vi "kpro 2016.vi"(0 "Output KPRO":path=path "c:/junk.dat", 1 "Initialize":bool, 2 "Finished In":bool, 3 "Cluster":T2, 5 "Absolute Depth In":sgl format="%.2f", 7 "Sensor Cluster In":T1, 11 "Flow":dbl format="%.2f", 12 "Read String Pot":bool, 13 "Increment":bool, 14 "SS In":i32) -> (4 "Finished Out":bool, 6 "SS Out":i32, 8 "Current Depth Out":sgl format="%.2f", 15 "Output Array":dbl[][](array[numeric])=[[17182499.0, -1.0, -1.0, 0.07295542423579193, 10.0, 30.0, 1.0, 0.2942041776993234, 33.989999999999995], [17194122.0, -2.0, -2.0, 0.08603630732168976, 10.0, 30.0, 1.0, 0.28579594169762795, 34.989999999999995], [17196835.0, -3.0, -3.0, 0.36859565057132326, 10.0, 30.0, 1.0, 0.27785495971103086, 35.989999999999995], [17198861.0, -4.0, -4.0, 0.493583415597236, 10.0, 30.0, 1.0, 0.27034333603676675, 36.989999999999995], [17203069.0, -5.0, -5.0, 0.23764258555133078, 10.0, 30.0, 1.0, 0.2632271650434325, 37.989999999999995], [17204351.0, -6.0, -6.0, 0.7800312012480499, 10.0, 30.0, 1.0, 0.2564760194921775, 38.989999999999995], [17205734.0, -7.0, -7.0, 0.7230657989877078, 10.0, 30.0, 1.0, 0.25006251562890724, 39.989999999999995], [17206879.0, -8.0, -8.0, 0.8733624454148472, 10.0, 30.0, 1.0, 0.24396194193705784, 40.989999999999995], [17208211.0, -9.0, -9.0, 0.7507507507507507, 10.0, 30.0, 1.0, 0.23815194093831868, 41.989999999999995], [17211804.0, -10.0, -10.0, 0.27831895352073477, 10.0, 30.0, 1.0, 0.23261223540358225, 42.989999999999995], [17214313.0, -11.0, -11.0, 0.3985651654045437, 10.0, 30.0, 1.0, 0.22732439190725168, 43.989999999999995], [17215593.0, -12.0, -12.0, 0.78125, 10.0, 30.0, 1.0, 0.22227161591464772, 44.989999999999995], [17216822.0, -13.0, -13.0, 0.8136696501220504, 10.0, 30.0, 1.0, 0.21743857360295718, 45.989999999999995], [17218103.0, -14.0, -14.0, 0.7806401249024201, 10.0, 30.0, 1.0, 0.2128112364332837, 46.989999999999995], [17219267.0, -15.0, -15.0, 0.859106529209622, 10.0, 30.0, 1.0, 0.20837674515524068, 47.989999999999995], [17220448.0, -16.0, -16.0, 0.8467400508044031, 10.0, 30.0, 1.0, 0.20412329046744235, 48.989999999999995], [17221627.0, -17.0, -17.0, 0.8481764206955046, 10.0, 30.0, 1.0, 0.20004000800160035, 49.989999999999995], [17222775.0, -18.0, -18.0, 0.8710801393728224, 10.0, 30.0, 1.0, 0.19611688566385568, 50.989999999999995], [17223888.0, -19.0, -19.0, 0.8984725965858041, 10.0, 30.0, 1.0, 0.19234468166955185, 51.989999999999995], [17225019.0, -20.0, -20.0, 0.8841732979664014, 10.0, 30.0, 1.0, 0.18871485185884132, 52.989999999999995], [17226151.0, -21.0, -21.0, 0.88339222614841, 10.0, 30.0, 1.0, 0.18521948508983146, 53.989999999999995], [17227282.0, -22.0, -22.0, 0.8841732979664014, 10.0, 30.0, 1.0, 0.18185124568103292, 54.989999999999995]] format="%.5f")   [LabVIEW 2016]
uses:
  controls/Kpro hydraulic measurement cluster.ctl
  controls/MCC DAQ Readings.ctl
  C:/Cascade-lv16-64/builds/Waterloo Main Program/cascade/data/ULx_LV.dll
  builds/Waterloo Main Program/cascade/data/ULx_LV.dll
panel:
  out "Sensor Cluster 2":T1
  in  "Sensor Cluster In 2":T1
  out "Array out":refnum<k24>[](array[refnum])
  in  "Array in":refnum<k24>[](array[refnum])
  in  "String Pot \nSlope 2":dbl=1.7339999675750732 format="%.2f"
  in  "error in (no error)":errorcluster
  in  "Descriptions":string[](array[string])
  in  "Output KPRO 2":path=path "c:/junk.dat"
  in  "Zeroed Pressure 2":dbl format="%.2f"
  out "Cluster Out":T2
  in  "String Pot \nSlope":dbl=1.7339999675750732 format="%.2f"
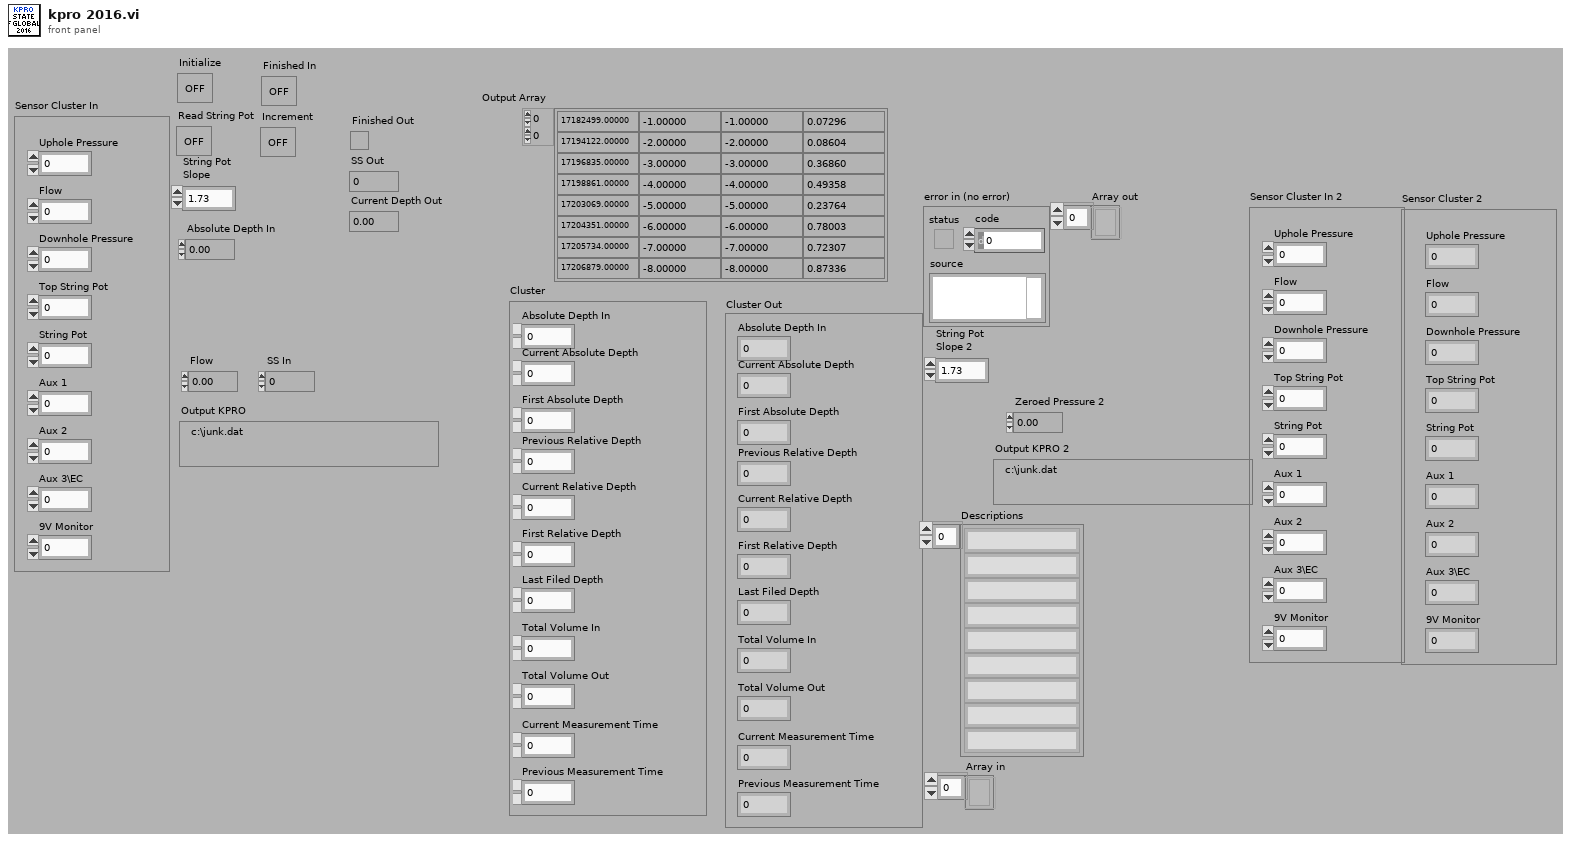
[diagram p1: front panel]
types:
  T1 = typedef "MCC DAQ Readings.ctl" = cluster{"Uphole Pressure":dbl, "Flow":dbl, "Downhole Pressure":dbl, "Top String Pot":dbl, "String Pot":dbl, "Aux 1":dbl, "Aux 2":dbl, "Aux 3\\EC":dbl, "9V Monitor":dbl}
  T2 = typedef "Kpro hydraulic measurement cluster.ctl" = cluster{"Absolute Depth In":dbl, "Current Absolute Depth":dbl, "First Absolute Depth":dbl, "Previous Relative Depth":dbl, "Current Relative Depth":dbl, "First Relative Depth":dbl, "Last Filed Depth":dbl, "Total Volume In":dbl, "Total Volume Out":dbl, "Current Measurement Time":dbl, "Previous Measurement Time":dbl}
  T3 = enum16{"Initialize", "Read", "Calc IK and generate Array", "Write Data & finish"}
  T4 = enum16{"Initialize", "Read", "read2", "Write Data & finish"}
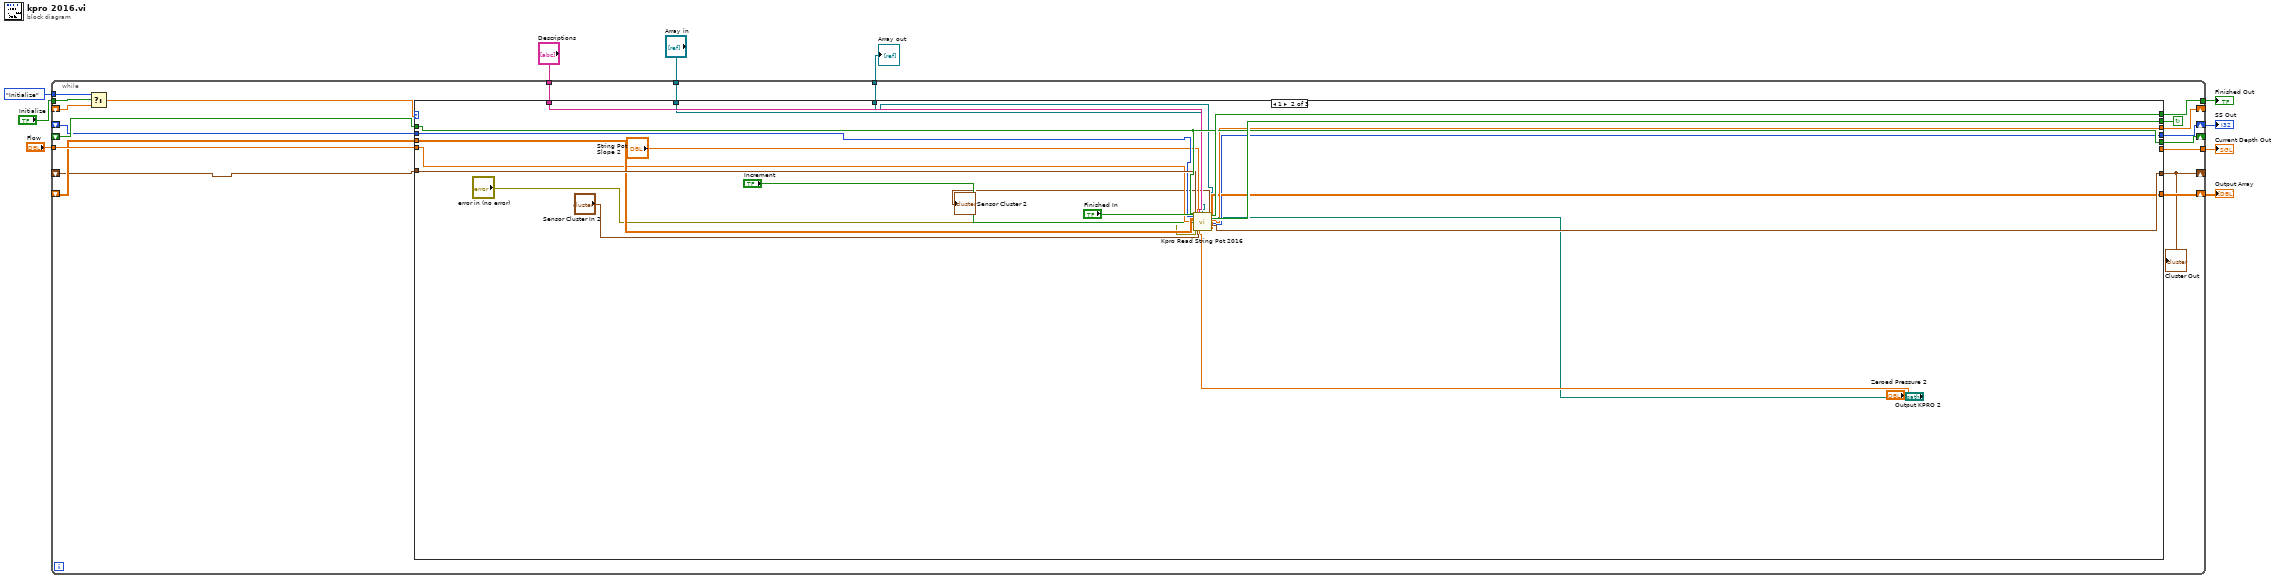
[diagram p0: block diagram]
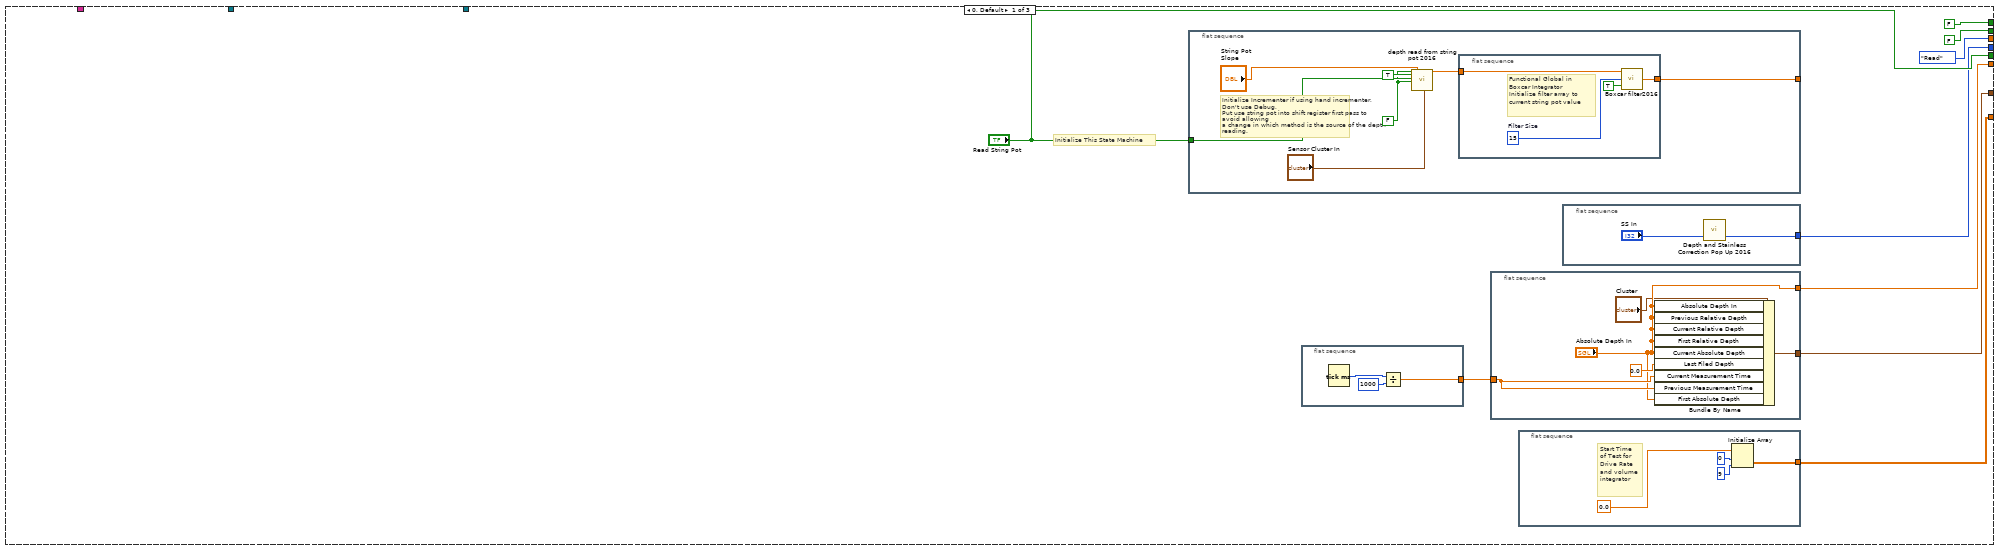
[diagram p2: hidden frame]
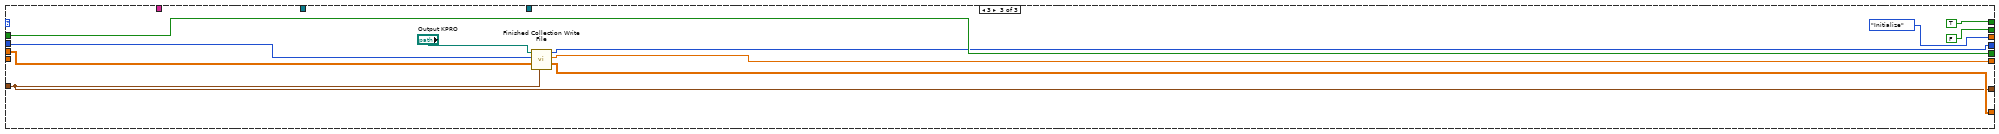
[diagram p3: hidden frame]
diagram:
  n1 = while {
    shift-left: _ -> [w22]
    shift-right: [w21] -> w5
    tunnel: [w23] -> w6
    tunnel: [w24] -> w7
    shift-left: _ -> [w25]
    shift-right: [w26] -> w4
    tunnel: "Flow" -> [w27]
    shift-left: _ -> [w28]
    shift-right: [w29] -> _
    tunnel: "Initialize" -> [w30]
    tunnel: T3."Initialize" -> [w19]
    shift-left: _ -> [w17]
    shift-right: [w16] -> _
    shift-right: [w15] -> _
    shift-left: _ -> [w14]
    tunnel: "Descriptions" -> [w13]
    tunnel: [w12] -> w2
    tunnel: "Array in" -> [w11]
    stop <- w20 continue-if-true
    n2 = Select(t=w19, s=w30, f=w17) -> (s? t:f=w18:dbl)
    n3 = case shown="1" w18 {
      tunnel: [T4."Read" w80 T3."Initialize"] -> w16
      tunnel: ["Read String Pot" w83 w96] -> w29
      tunnel: w28 -> [_ w83 w96]
      tunnel: w27 -> [_ w76 _]
      tunnel: [w38 w78 w93] -> w26
      tunnel: w25 -> [_ w79 w95]
      tunnel: [w31 _ w94] -> w24
      tunnel: [FALSE w86 FALSE] -> w20
      tunnel: [FALSE w84 TRUE] -> w23
      tunnel: w22 -> [_ w77 w91]
      tunnel: [w35 w75 w90] -> w21
      tunnel: [w33 w81 w88] -> w15
      tunnel: w14 -> [_ w82 w88]
      tunnel: w13 -> [_ w74 _]
      tunnel: [_ w73 _] -> w12
      tunnel: w11 -> [_ w72 _]
      frame 0, Default {
        # "Initialize This State Machine"
        n4 = flat-sequence {
          tunnel: "Read String Pot" -> [w54]
          tunnel: [w52] -> _
          frame #0 {
            w53 = FALSE
            # "Initialize Incrementer if using hand incrementer,\nDon't use Debug,\nPut use string pot into shift register first pass to avoid allowing\na change in which method is the source of the depth reading."
            n5 = call "depth read from string pot 2016.vi"(0:w53, 1:TRUE, 2:w54, 3:w53, "String Pot \nSlope"="String Pot \nSlope", "Sensor Cluster In"="Sensor Cluster In") -> ("Depth"=w56:dbl)  [unwired: 10 in, 3 out]
            n6 = flat-sequence {
              tunnel: w56 -> [w58]
              tunnel: [w57] -> w52
              frame #0 {
                w59 = 15  # Filter Size
                # "Functional Global in \nBoxcar Integrator\nInitialize filter array to \ncurrent string pot value"
                n7 = call "Boxcar filter2016.vi"("Initialize"=TRUE, "Filter Size"=w59, "Filter Input"=w58) -> ("Filter Output"=w57:dbl)
              }
            }
          }
        }
        n8 = flat-sequence {
          tunnel: [w47] -> w32
          frame #0 {
            n9 = Tick Count (ms)() -> (millisecond timer value=w49:u32)
            n10 = Divide(x=w49, y=u32 1000) -> (x/y=w47:dbl)
          }
        }
        n11 = flat-sequence {
          tunnel: [w46] -> w33
          tunnel: w32 -> [w44]
          tunnel: ["Absolute Depth In"] -> w31
          frame #0 {
            n12 = Bundle By Name(cluster="Cluster", "Absolute Depth In"="Absolute Depth In", "Previous Relative Depth"="Absolute Depth In", "Current Relative Depth"="Absolute Depth In", "First Relative Depth"="Absolute Depth In", "Current Absolute Depth"="Absolute Depth In", "Last Filed Depth"=0.0, "Current Measurement Time"=w44, "Previous Measurement Time"=w44, "First Absolute Depth"="Absolute Depth In") -> (w46:T2)
          }
        }
        n13 = flat-sequence {
          tunnel: [w64] -> w38
          frame #0 {
            # "Start Time\nof Test for\nDrive Rate\nand volume\nintegrator"
            n14 = Initialize Array(0.0, 0, 9) -> (w64:dbl[][])
          }
        }
        n15 = flat-sequence {
          tunnel: [w40] -> w35
          frame #0 {
            n16 = call "Depth and Stainless Correction Pop Up 2016.vi"("New Number\n of Stainless\n(Count)"="SS In") -> ("Feet of\nStainless to be\nUsed (Count)"=w40:i32)  [unwired: 1 in, 1 out]
          }
        }
      }
      frame 1 {
        n17 = call "Kpro Read String Pot 2016.vi"("Read String Pot"=w83, "Feet of\nStainless to be\nUsed (Count) in"=w77, "Session Array in"=w79, "Flow"=w76, "Manual Depth In"="Increment", "Finished In"="Finished In", "Depth Cluster in"=w82, "error in (no error)"="error in (no error)", "String Pot \nSlope in"="String Pot \nSlope 2", "Sensor Cluster In in"="Sensor Cluster In 2", "Descriptions"=w74, "Pressure in"="Zeroed Pressure 2", "Array in"=w72, "Initial Measurement Input"="Output KPRO 2") -> ("Sensor Cluster 2"=→"Sensor Cluster 2":T1, "Array out"=w73:refnum<k24>[], "Generate Array Calc IK"=w84:bool, "Finish Take Data"=w86:bool, "Depth Rate"=w80:dbl, "Feet of\nStainless to be\nUsed (Count) out"=w75:i32, "Depth Cluster out"=w81:T2, "Single String Pot Session Array out"=w78:dbl[][])  [unwired: 3 in, 3 out]
      }
      frame 3 {
        n18 = call "Finished Collection Write File.vi"("Cluster in"=w88, "Corrected Array in"=w95, "Feet of\nStainless to be\nUsed (Count) in"=w91, "Output KPRO"="Output KPRO") -> ("Corrected Array out"=w93:dbl[][], "Depth to \nbe Used \n(Feet)"=w94:sgl, "Feet of\nStainless to be\nUsed (Count) out"=w90:i32)  [unwired: 5 in]
      }
    }
    "Cluster Out" <- w15
  }
  "Current Depth Out" <- w7
  "Finished Out" <- w6
  "SS Out" <- w5
  "Output Array" <- w4
  "Array out" <- w2
